vi "Channel.BuildMenuNames.vi"(11 "Aliases":T1[](array[typedef])) -> (3 "Aliases Array":string[](array[string]))   [LabVIEW 2013, in "Simple Sequence Tools - Shared.lvlib"]
uses:
  Simple Sequence Tools - Shared.lvlib
  Types/Channel.Properties.ctl
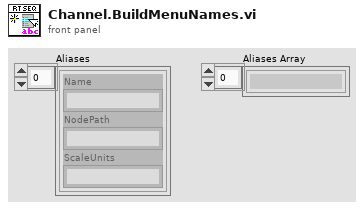
[diagram p1: front panel]
types:
  T1 = typedef "Simple Sequence Tools - Shared.lvlib/Channel.Properties.ctl" = cluster{"Name":string, "NodePath":string, "ScaleUnits":string}
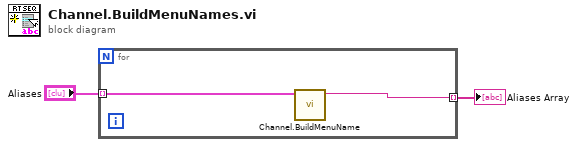
[diagram p0: block diagram]
diagram:
  n1 = for {
    tunnel: "Aliases" -> [w4] mode=indexing
    tunnel: [w3] -> w2 mode=indexing
    n2 = call "Channel.BuildMenuName.vi"("cluster"=w4) -> ("NodePath"=w3:string)  [unwired: 10 in]
  }
  "Aliases Array" <- w2
